vi "加工.vi"(8 "error in (no error)":errorcluster caption="错误输入（无错误）", 11 "铣削 输入":refnum<class "铣削.lvclass"> caption="DNL_LabVIEW Object in") -> (0 "error out":errorcluster caption="错误输出", 3 "铣削 输出":refnum<class "铣削.lvclass"> caption="DNL_LabVIEW Object out")   [LabVIEW 2011, in "铣削.lvclass"]
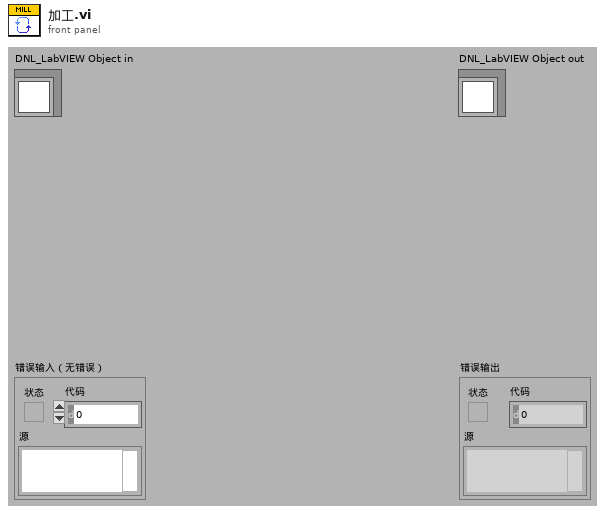
[diagram p1: front panel]
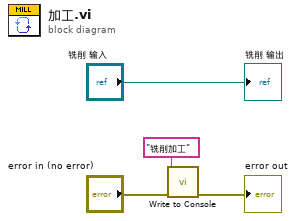
[diagram p0: block diagram]
diagram:
  n1 = call "Write to Console.vi"("error in (no error)"="error in (no error)", "Input"="铣削加工") -> ("error out"=→"error out":errorcluster)  [unwired: 9 in]
  "铣削 输出" <- "铣削 输入"
